vi "TW Post-Project-Copying Process - Stage 3.vi"(8 "error in":errorcluster, 10 "New Subname":string, 11 "Template Project Path":path) -> (0 "error out":errorcluster)   [LabVIEW 2021, in "Plugin Generator.lvlib"]
uses:
  Plugin Generator.lvlib
  <vilib>/CIF Foundation/CIF LabVIEW Scripting/LV Scripting/LV Scripting Utilities.lvlib
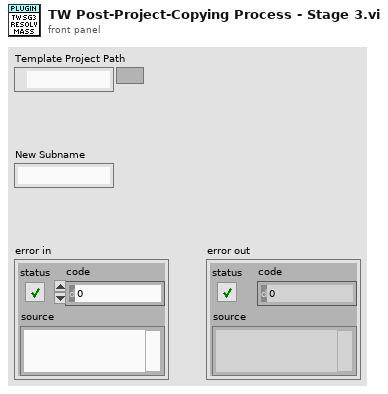
[diagram p1: front panel]
types:
  T1 = typedef "Edit LVProj.lvlib/Library And VI References.ctl" = cluster{"Target Reference":refnum<vi>, "VI References":refnum<vi>[], "Library References":refnum<vi>[]}
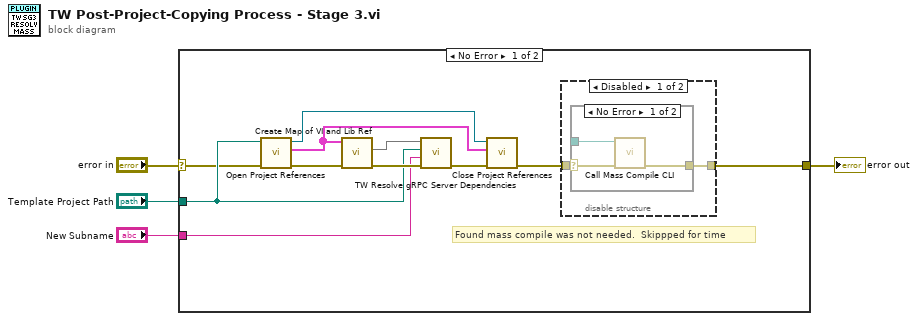
[diagram p0: block diagram]
diagram:
  n1 = case shown="No Error" "error in" {
    selector: "error in" -> [w10 w23]
    tunnel: [w15 w23] -> w4
    tunnel: "New Subname" -> [w12 _]
    tunnel: "Template Project Path" -> [w11 _]
    frame No Error {
      # "Found mass compile was not needed.  Skippped for time"
      n2 = call <vilib>:"Open Project References.vi"("error in"=w10, "Project Path"=w11) -> ("error out"=w9:errorcluster, "VI and Library References"=w5:T1[], "Project Reference"=w7:refnum<vi>)  [unwired: 7 in]
      n3 = call <vilib>:"Create Map of VI and Lib Ref.vi"("error in"=w9, "VI and Library References"=w5) -> ("error out"=w13:errorcluster, "Library Map"=w14:map{string, refnum<vi>})  [unwired: 7 in, 1 out]
      n4 = call "TW Resolve gRPC Server Dependencies.vi"("error in"=w13, "New Subname"=w12, "Template Project Path"=w11, "Map - LibRef"=w14) -> ("error out"=w8:errorcluster)  [unwired: 7 in]
      n5 = call <vilib>:"Close Project References.vi"("error in"=w8, "VI and Library References"=w5, "Project Reference"=w7) -> ("error out"=w6:errorcluster)  [unwired: 8 in]
      n6 = disable-structure shown="Disabled" {
        disable-tunnel: [w17 w22] -> w15
        disable-tunnel: w6 -> [w16 w22]
        frame Disabled {
          n7 = case shown="No Error" w16 {
            selector: w16 -> [w19 w21]
            tunnel: [w18 w21] -> w17
            tunnel: _ -> [w20 _]
            frame No Error {
              n8 = call <vilib>:"Call Mass Compile CLI.vi"("error in"=w19, "Directory"=w20) -> ("error out"=w18:errorcluster)  [unwired: 9 in]
            }
            frame Error {
            }
          }
        }
        frame Enabled {
        }
      }
    }
    frame Error {
    }
  }
  "error out" <- w4
